vi "AlphaBetaToABC_UnitaryMagnitude_src.vi"(0 "alpha":sgl, 5 "beta":sgl) -> (4 "A":sgl, 6 "B":sgl, 8 "C":sgl)   [LabVIEW 2015]
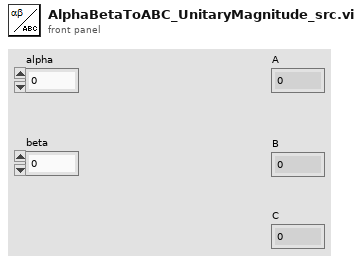
[diagram p1: front panel]
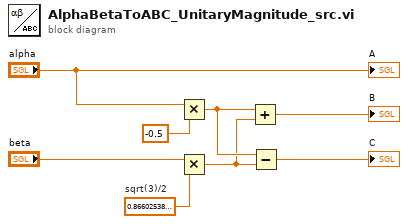
[diagram p0: block diagram]
diagram:
  w1 = sgl 0.8660254  # sqrt(3)/2
  n1 = Multiply(x="alpha", y=sgl -0.5) -> (x*y=w7:sgl)
  n2 = Multiply(x="beta", y=w1) -> (x*y=w6:sgl)
  n3 = Add(x=w7, y=w6) -> (x+y=→"B":sgl)
  n4 = Subtract(x=w7, y=w6) -> (x-y=→"C":sgl)
  "A" <- "alpha"
